vi "UnloadPanel.vi"(8 "error in (no error)":errorcluster caption="entrée d'erreur (pas d'erreur)", 11 "Device en entrée":refnum<class "BaseDevice.lvclass"> caption="DNL_LabVIEW Object in") -> (0 "error out":errorcluster caption="sortie d'erreur", 3 "Device en sortie":refnum<class "BaseDevice.lvclass"> caption="DNL_LabVIEW Object out")   [LabVIEW 2019, in "BaseDevice.lvclass"]
uses:
  BaseDevice.lvclass
  BaseDevice.lvclass/BaseDevice.ctl
  ClassQueueMess.ctl
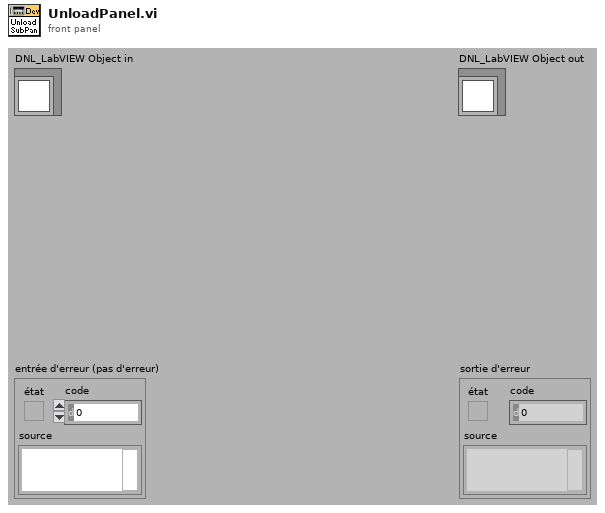
[diagram p1: front panel]
types:
  T1 = enum32{"Bad", "Idle", "Run top level", "Running"}
  T2 = typedef "ClassQueueMess.ctl" = u16
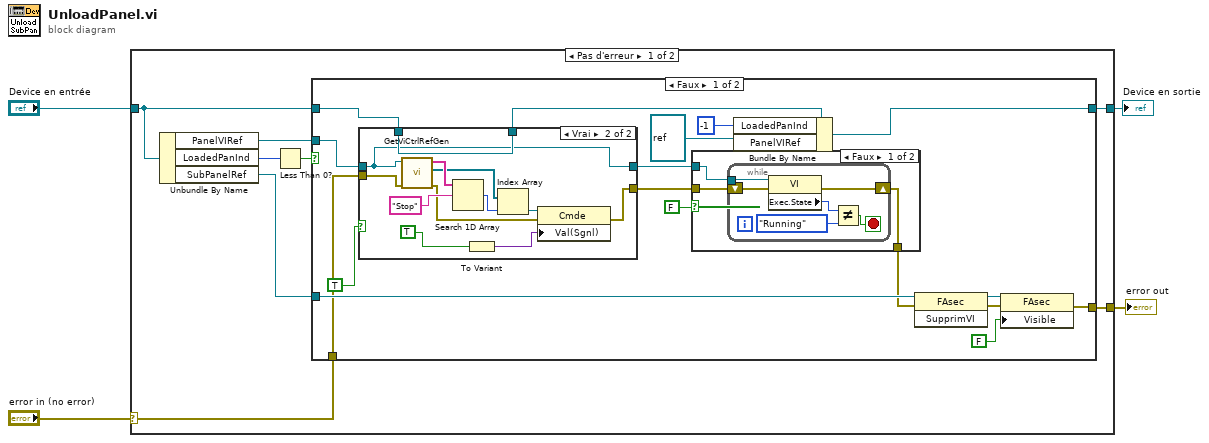
[diagram p0: block diagram]
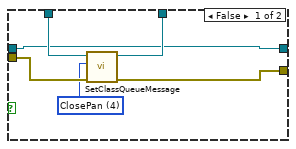
[diagram p2: hidden frame]
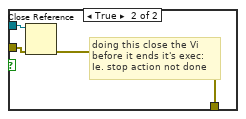
[diagram p3: hidden frame]
diagram:
  n1 = case shown="Pas d'erreur" "error in (no error)" {
    selector: "error in (no error)" -> [w11 w63]
    tunnel: [w10 w63] -> w3
    tunnel: [w8 w62] -> w1
    tunnel: "Device en entrée" -> [w9 w62]
    frame No Error {
      n2 = Unbundle By Name(w9) -> ("PanelVIRef"=w12:refnum<vi>, "LoadedPanInd"=w7:i32, "SubPanelRef"=w5:refnum<vi>)
      n3 = Less Than 0?(x=w7) -> (x < 0?=w6:bool)
      n4 = case shown="Faux" w6 {
        tunnel: w12 -> [w17 _]
        tunnel: w11 -> [w18 w60]
        tunnel: [w21 w60] -> w10
        tunnel: w9 -> [w14 w61]
        tunnel: [w26 w61] -> w8
        tunnel: w5 -> [w24 _]
        frame False {
          n5 = case shown="Vrai" TRUE ("Booléen") {
            tunnel: [w32 w37] -> w29
            tunnel: [w30 w36] -> w28
            tunnel: w18 -> [w33 w46]
            tunnel: w17 -> [w30 w36]
            tunnel: w14 -> [w35 w47]
            tunnel: [w34 w47] -> w15
            frame False {
              w31 = T2 4 items=["UpdateClassData", "UpdateMainClass", "UpdateDataBind", "ReInitDevice", "ClosePan"] ("Menu déroulant")
              n6 = call-dynamic "SetClassQueueMessage.vi"("ErrorIn(No Error)"=w33, "Menu déroulant"=w31, "BaseDevice.lvclass"=w35) -> ("sortie d'erreur"=w32:errorcluster, "BaseDevice.lvclass Out"=w34:refnum<class "BaseDevice.lvclass">)  [unwired: 7 in]
            }
            frame True {
              n7 = call <userlib>:"GetViCtrlRefGen.vi"("ErrorIn(No Error)"=w46, "VIRef"=w36) -> ("sortie d'erreur"=w40:errorcluster, "ControlsRefs"=w43:refnum<vi>[], "ControlsNames"=w45:string[])  [unwired: 7 in]
              n8 = Search 1D Array(1D array=w45, element="Stop" ("Nom de la commande")) -> (index of element=w42:i32)  [unwired: 1 in]
              n9 = To Variant(anything=TRUE) -> (Variant=w38:variant)
              n10 = Index Array(array=w43, index=w42) -> (element=w41:refnum<vi>)
              n11 = property class="Cmde"(reference=w41, error in=w40, "Val(Sgnl)"=w38) -> (error out=w37:errorcluster)  [unwired: 1 out]
            }
          }
          n12 = case shown="Faux" FALSE {
            tunnel: w29 -> [w49 w59]
            tunnel: w28 -> [w50 w58]
            tunnel: [w48 w57] -> w23
            frame False {
              n13 = while {
                tunnel: w50 -> [w56]
                shift-right: [w54] -> w48
                shift-left: w49 -> [w55]
                stop <- w51 stop-if-true
                n14 = property class="VI"(reference=w56, error in=w55) -> (error out=w54:errorcluster, "Exec.State"=w52:T1)  [unwired: 1 out]
                n15 = Not Equal?(x=w52, y=T1."Running" ("Exécution:État")) -> (x != y?=w51:bool)
              }
            }
            frame True {
              # "doing this close the Vi before it ends it's exec:\nIe. stop action not done"
              n16 = Close Reference(reference=w58, error in (no error)=w59) -> (error out=w57:errorcluster)
            }
          }
          n17 = Bundle By Name(cluster=w15, "LoadedPanInd"=-1 ("LoadedPanelIndex"), "PanelVIRef"=refnum<vi> refnum ("StatPanelRef")) -> (w26:refnum<class "BaseDevice.lvclass">)
          n18 = invoke class="FAsec" method="SupprimVI"(reference=w24, error in=w23) -> (reference out=w20:refnum<vi>, error out=w19:errorcluster)  [unwired: 1 in, 1 out]
          n19 = property class="FAsec"(reference=w20, error in=w19, "Visible"=FALSE) -> (error out=w21:errorcluster)  [unwired: 1 out]
        }
        frame True {
        }
      }
    }
    frame Error {
    }
  }
  "error out" <- w3
  "Device en sortie" <- w1
